vi "parse field names from SELECT statement.vi"(1 "Select String":string="select method_ident , \nparent_tag , \nchild_tag , \nchild_position , \nchild_label , \nchild_value , \nrevision_nbr \nfrom change_stack\nwhere 1=0") -> (0 "variant(field names)":variant[](array[variant]))   [LabVIEW 2020, in "hse-db-ado.lvlib" / "ADO-DB-Driver.lvlib"]
doc: "Parse a select statement into an array of variant fields\n\n____\nHAMPEL SOFTWARE ENGINEERING v1.4.0 (2023-12-19 09:52)"
uses:
  ADO-DB-Driver.lvlib
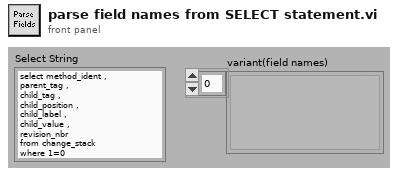
[diagram p1: front panel]
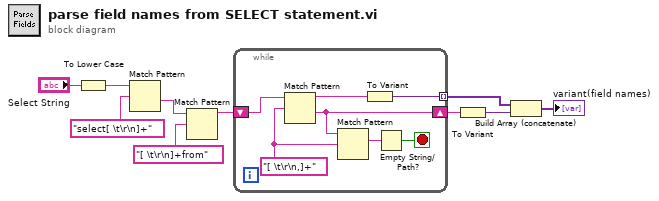
[diagram p0: block diagram]
diagram:
  n1 = To Lower Case(string="Select String") -> (all lower case string=w1:string)
  n2 = Match Pattern(string=w1, regular expression="select[ \t\r\n]+") -> (after substring=w8:string)  [unwired: 1 in, 3 out]
  n3 = Match Pattern(string=w8, regular expression="[ \t\r\n]+from") -> (before substring=w6:string)  [unwired: 1 in, 3 out]
  n4 = while {
    shift-right: [w15] -> w3
    shift-left: w6 -> [w17]
    tunnel: [w11] -> w5 mode=indexing
    stop <- w13 stop-if-true
    w16 = "[ \t\r\n,]+" ("regular expression")
    n5 = Match Pattern(string=w17, regular expression=w16) -> (before substring=w12:string, after substring=w15:string)  [unwired: 1 in, 2 out]
    n6 = Match Pattern(string=w15, regular expression=w16) -> (match substring=w14:string)  [unwired: 1 in, 3 out]
    n7 = To Variant(anything=w12) -> (Variant=w11:variant)
    n8 = Empty String/Path?(string/path=w14) -> (empty?=w13:bool)
  }
  n9 = To Variant(anything=w3) -> (Variant=w2:variant)
  n10 = Build Array (concatenate)(w5, w2) -> (→"variant(field names)":variant[])
